vi "Parse Register Message.vi"(0 "state":string, 1 "Module Name":string, 5 "args":string) -> (4 "target":string, 6 "source":string, 8 "status":string, 10 "api":string)   [LabVIEW 2020, in "Communicable State Machine.lvlib"]
uses:
  Communicable State Machine.lvlib
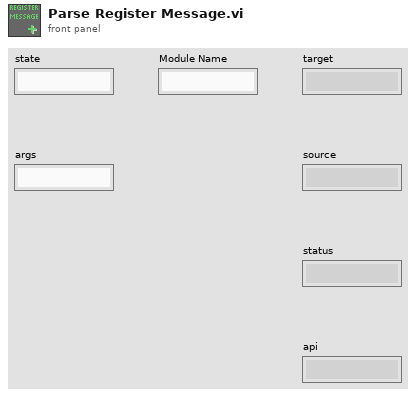
[diagram p1: front panel]
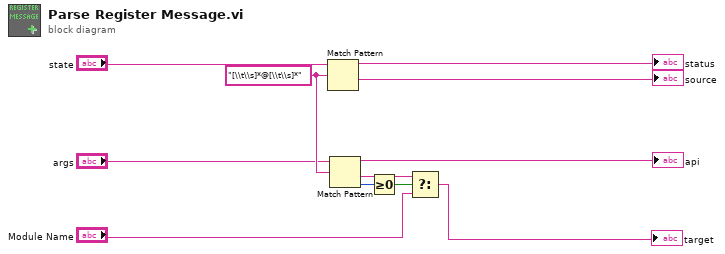
[diagram p0: block diagram]
diagram:
  w8 = "[\\t\\s]*@[\\t\\s]*" ("regular expression")
  n1 = Match Pattern(string="state", regular expression=w8) -> (before substring=→"status":string, after substring=→"source":string)  [unwired: 1 in, 2 out]
  n2 = Match Pattern(string="args", regular expression=w8) -> (before substring=→"api":string, after substring=w9:string, offset past match=w11:i32)  [unwired: 1 in, 1 out]
  n3 = Greater Or Equal To 0?(x=w11) -> (x >= 0?=w10:bool)
  n4 = Select(t=w9, s=w10, f="Module Name") -> (s? t:f=→"target":string)
